vi "Long sweep.vi"() -> (1 "Channel Names":string[](array[string]), 2 "Sequence out":refnum<class "Sequence Config.lvclass">)   [LabVIEW 2018, in "Sequencer Module tests.lvlib"]
uses:
  Sequencer Module tests.lvlib
  classes/Sequence/Config/Sequence Config.lvclass
  basic steps/Wait Step/Config/Wait Step Config.lvclass
  C:/Git/DCAF-Sequencer-Module/Prototype/classes/Step/Config/Step Config.lvclass
  <vilib>/NI/Tag Bus/tag/Data Type.ctl
  basic steps/Update Tag Step/Config/Update Tag Configuration/Update Tag Config.lvclass
  <vilib>/NI/Tag Bus Module Framework/channel/channel classification.ctl
  <vilib>/NI/Tag Bus/tag/tag descriptor.lvclass/tag descriptor.ctl
  <vilib>/NI/Tag Bus Module Framework/channel/TBM channel.lvclass
  C:/Program Files (x86)/National Instruments/LabVIEW 2018/vi.lib/NI/Tag Bus/tag/tag descriptor.lvclass
  classes/Step/Config/Step Config.lvclass
  <vilib>/NI/Tag Bus/tag/tag descriptor.lvclass
panel:
  in  "Tag Name 1":string="Boolean processing result 0"
  in  "Name":string="Led Sequence"
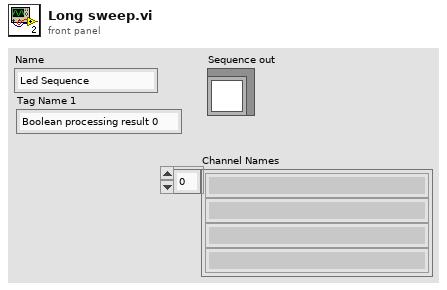
[diagram p1: front panel]
types:
  T1 = typedef "TBM channel.lvclass/channel classification.ctl" = enum16{"input data", "output data", "processing parameter", "processing result"}
  T2 = typedef "tag bus.lvlib/tag descriptor.lvclass/Data Type.ctl" = enum16{"Double", "Single", "I64", "I32", "I16", "I8", "U64", "U32", "U16", "U8", "Boolean", "String", "Array of Double", "Array of Single", "Array of I64", "Array of I32", "Array of I16", "Array of I8", "Array of U64", "Array of U32", "Array of U16", "Array of U8", "Array of Boolean", "Array of String"}
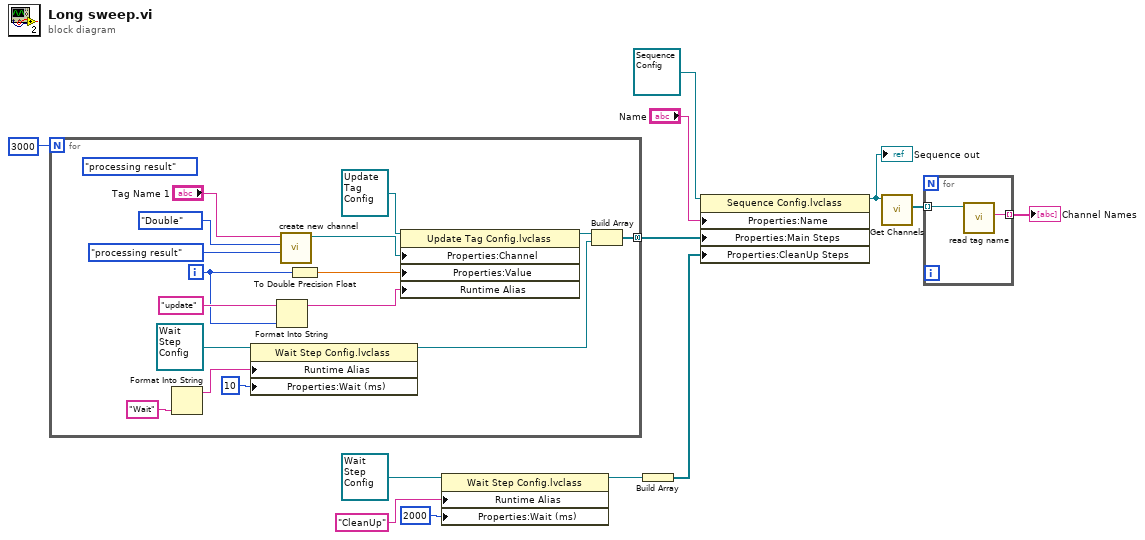
[diagram p0: block diagram]
diagram:
  n1 = for {
    N: 3000 -> [_]
    tunnel: [w28] -> w12 mode=concatenating
    i -> [w15]
    (unwired) channel_classification."processing result" ("channel classification")
    n2 = Format Into String("Wait" ("Runtime Alias")) -> (resulting string=w14:string)  [unwired: 3 in, 1 out]
    n3 = property class="Wait Step Config.lvclass"(reference=refnum<class "Wait Step Config.lvclass"> refnum ("Wait Step Config.lvclass"), "Runtime Alias"=w14, "Properties:Wait (ms)"=u32 10 ("Wait (ms)")) -> (reference out=w19:refnum<class "Wait Step Config.lvclass">)  [unwired: 1 in, 1 out]
    n4 = Format Into String(initial string="update" ("Runtime Alias"), w15) -> (resulting string=w16:string)  [unwired: 2 in, 1 out]
    n5 = call <vilib>:"create new channel.vi"("channel classification"=channel_classification."processing result", "data type"=Data_Type."Double" ("Data Type"), "channel name"="Tag Name 1") -> ("channel"=w24:refnum<class "TBM channel.lvclass">)  [unwired: 8 in]
    n6 = To Double Precision Float(number=w15) -> (double precision float=w18:dbl)
    n7 = property class="Update Tag Config.lvclass"(reference=refnum<class "Update Tag Config.lvclass"> refnum ("Update Tag Config.lvclass"), "Properties:Channel"=w24, "Properties:Value"=w18, "Runtime Alias"=w16) -> (reference out=w22:refnum<class "Update Tag Config.lvclass">)  [unwired: 1 in, 1 out]
    n8 = Build Array(w22, w19) -> (w28:refnum<class "Step Config.lvclass">[])
  }
  n9 = property class="Wait Step Config.lvclass"(reference=refnum<class "Wait Step Config.lvclass"> refnum ("Wait Step Config.lvclass"), "Runtime Alias"="CleanUp", "Properties:Wait (ms)"=u32 2000 ("Wait (ms)")) -> (reference out=w7:refnum<class "Wait Step Config.lvclass">)  [unwired: 1 in, 1 out]
  n10 = Build Array(w7) -> (w6:refnum<class "Wait Step Config.lvclass">[])
  n11 = property class="Sequence Config.lvclass"(reference=refnum<class "Sequence Config.lvclass"> refnum ("Sequence Config.lvclass"), "Properties:Name"="Name", "Properties:Main Steps"=w12, "Properties:CleanUp Steps "=w6) -> (reference out=w2:refnum<class "Sequence Config.lvclass">)  [unwired: 1 in, 1 out]
  "Sequence out" <- w2
  n12 = call "Get Channels.vi"("Sequence Config in"=w2) -> ("Channels"=w4:refnum<class "TBM channel.lvclass">[])  [unwired: 8 in, 2 out]
  n13 = for {
    tunnel: w4 -> [w30] mode=indexing
    tunnel: [w29] -> w3 mode=indexing
    n14 = call <vilib>:"read tag name.vi"("system tag in"=w30) -> ("name"=w29:string)  [unwired: 8 in, 2 out]
  }
  "Channel Names" <- w3
